vi "Send Recieve Request for Result.vi"(6 "Request time":timestamp, 7 "Message Priority (Normal)":T1=enum."Normal", 8 "error in (no error)":errorcluster, 9 "Requestor":string, 10 "Requestee":string, 11 "Message Enqueuer":refnum<class "Message Enqueuer.lvclass">) -> (0 "error out":errorcluster, 3 "Message Enqueuer out":refnum<class "Message Enqueuer.lvclass">)   [LabVIEW 2015, in "Recieve Request for Result Msg.lvclass"]
doc: "This VI sends the message to an actor."
uses:
  Recieve Request for Result Msg.lvclass
  <vilib>/ActorFramework/Message Enqueuer/Message Enqueuer.lvclass
  <vilib>/ActorFramework/Message Enqueuer/Message Priority.ctl
  Recieve Request for Result Msg.lvclass/Recieve Request for Result Msg.ctl
  <vilib>/ActorFramework/Message Enqueuer/Message Enqueuer.lvclass/Message Enqueuer.ctl
  <vilib>/ActorFramework/Message Priority Queue/Priority Enqueue.vi
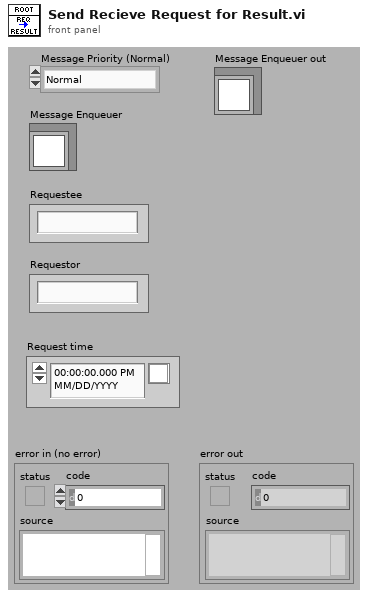
[diagram p1: front panel]
types:
  T1 = typedef "Actor Framework.lvlib/Message Enqueuer.lvclass/Message Priority.ctl" = enum16{"Low", "Normal", "High"}
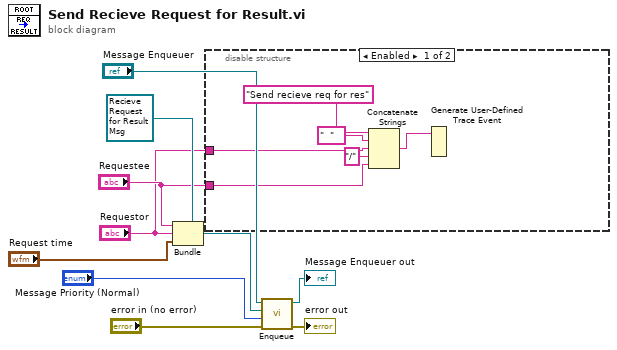
[diagram p0: block diagram]
diagram:
  n1 = Bundle(cluster=refnum<class "Recieve Request for Result Msg.lvclass"> refnum ("Object"), "Requestee", "Requestor", "Request time") -> (w6:refnum<class "Recieve Request for Result Msg.lvclass">)
  n2 = disable-structure shown="Enabled" {
    disable-tunnel: "Requestee" -> [w12 _]
    disable-tunnel: "Requestor" -> [w15 _]
    frame Enabled {
      n3 = Concatenate Strings("Send recieve req for res" ("string"), "  " ("string"), w15, "/" ("string"), w12) -> (w11:string)
      n4 = Generate User-Defined Trace Event(2:w11) -> ()  [unwired: 1 in]
    }
    frame Disabled {
    }
  }
  n5 = call <vilib>:"Enqueue.vi"("error in (no error)"="error in (no error)", "Message Priority (Normal)"="Message Priority (Normal)", "Message"=w6, "Message Enqueuer in"="Message Enqueuer") -> ("error out"=→"error out":errorcluster, "Message Enqueuer out"=→"Message Enqueuer out":refnum<class "Message Enqueuer.lvclass">)  [unwired: 6 in]
